vi "Find Lines.vi"(8 "error in":errorcluster, 11 "Image In":T1) -> (0 "error out":errorcluster, 1 "XY Graph":cluster{dbl[], dbl[]}(graph), 2 "Lines Calibrated (Shape Detection 1)":T2(array[cluster]) {"End Point"."Y" format="%.2f"; "End Point"."X" format="%.2f"; "Start Point"."Y" format="%.2f"; "Start Point"."X" format="%.2f"}, 3 "Image Out":T1)   [LabVIEW 2012]
uses:
  <vilib>/vision/Image Controls.llb/IMAQ Image.ctl
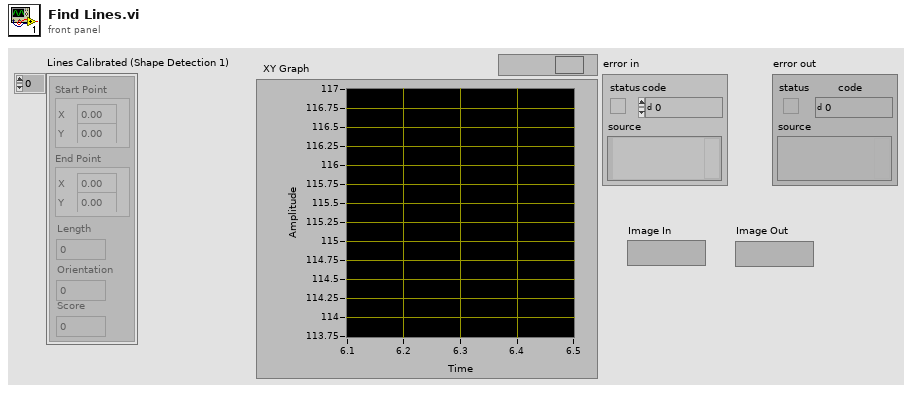
[diagram p1: front panel]
types:
  T1 = typedef "IMAQ Image.ctl" = refnum<image>
  T2 = cluster{"Start Point":cluster{"X":sgl, "Y":sgl}, "End Point":cluster{"X":sgl, "Y":sgl}, "Length":dbl, "Orientation":dbl, "Score":dbl}[]
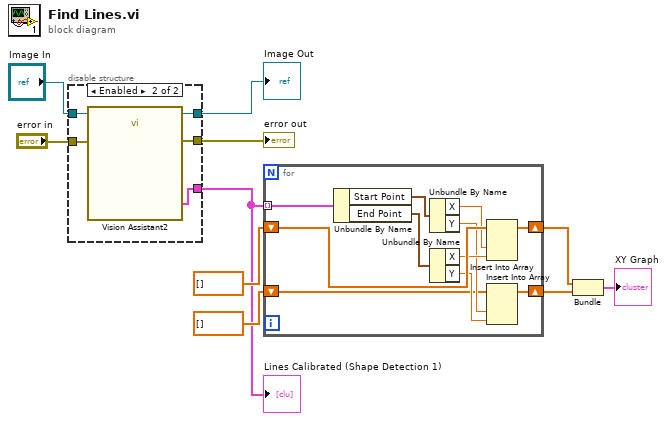
[diagram p0: block diagram]
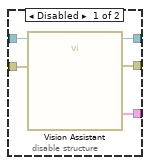
[diagram p2: hidden frame]
diagram:
  n1 = disable-structure shown="Enabled" {
    disable-tunnel: [w15 w20] -> w10
    disable-tunnel: [w14 w16] -> w4
    disable-tunnel: "Image In" -> [w13 w17]
    disable-tunnel: "error in" -> [w12 w18]
    disable-tunnel: [w11 w19] -> w1
    frame Disabled {
      n2 = call "Vision Assistant"("Image In"=w13, "error in"=w12) -> ("Image Out"=w15:T1, "Lines Calibrated (Shape Detection 1)"=w14:T2, "error out"=w11:errorcluster)  [unwired: 22 in, 1 out]
    }
    frame Enabled {
      n3 = call "Vision Assistant2"("Image In"=w17, "error in"=w18) -> ("Image Out"=w20:T1, "Lines Calibrated (Shape Detection 1)"=w16:T2, "error out"=w19:errorcluster)  [unwired: 22 in, 1 out]
    }
  }
  "Image Out" <- w10
  "Lines Calibrated (Shape Detection 1)" <- w4
  "error out" <- w1
  n4 = for {
    tunnel: w4 -> [w31] mode=indexing
    shift-right: [w23] -> w6
    shift-left: dbl[] [] -> [w30]
    shift-right: [w21] -> w5
    shift-left: dbl[] [] -> [w22]
    n5 = Unbundle By Name(w31) -> ("Start Point"=w28:cluster{"X":sgl, "Y":sgl}, "End Point"=w29:cluster{"X":sgl, "Y":sgl})
    n6 = Unbundle By Name(w28) -> ("X"=w27:sgl, "Y"=w25:sgl)
    n7 = Unbundle By Name(w29) -> ("X"=w26:sgl, "Y"=w24:sgl)
    n8 = Insert Into Array(array=w30, new element #1=w27, new element #2=w26) -> (w23:dbl[])  [unwired: 1 in]
    n9 = Insert Into Array(array=w22, new element #1=w25, new element #2=w24) -> (w21:dbl[])  [unwired: 1 in]
  }
  n10 = Bundle(w6, w5) -> (→"XY Graph":cluster{dbl[], dbl[]})  [unwired: 1 in]
